vi "Has all samples.vi"(8 "error in (no error)":errorcluster, 11 "Automatic Mode in":refnum<class "Automatic Mode.lvclass">) -> (0 "error out":errorcluster, 2 "Has all samples?":bool, 3 "Automatic Mode out":refnum<class "Automatic Mode.lvclass">)   [LabVIEW 2015, in "Automatic Mode.lvclass"]
uses:
  Automatic Mode.lvclass
  Automatic Mode.lvclass/Automatic Mode.ctl
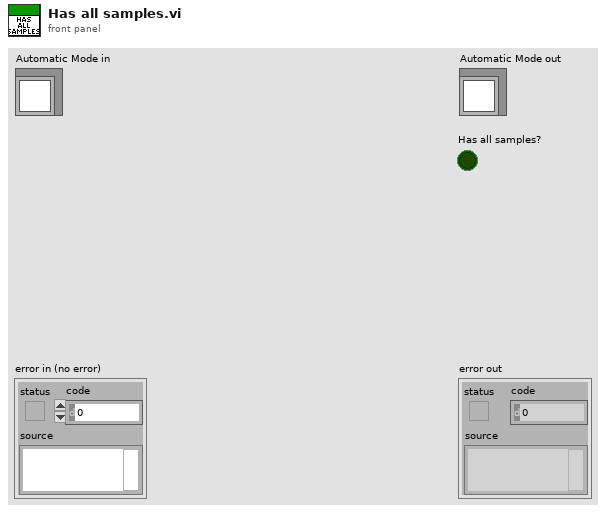
[diagram p1: front panel]
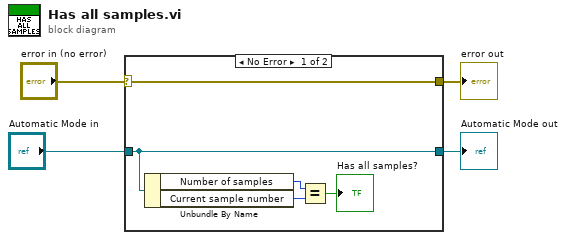
[diagram p0: block diagram]
diagram:
  n1 = case shown="No Error" "error in (no error)" {
    selector: "error in (no error)" -> [w9 w11]
    tunnel: [w9 w11] -> w3
    tunnel: [w8 w10] -> w1
    tunnel: "Automatic Mode in" -> [w8 w10]
    frame No Error {
      n2 = Unbundle By Name(w8) -> ("Number of samples"=w7:i32, "Current sample number"=w6:i32)
      n3 = Equal?(x=w7, y=w6) -> (x = y?=→"Has all samples?":bool)
    }
    frame Error {
    }
  }
  "error out" <- w3
  "Automatic Mode out" <- w1
